vi "Check For Stop.vi"(8 "error in (no error)":errorcluster, 10 "local stop (F)":bool, 11 "User Interface in":refnum<class "User Interface.lvclass">) -> (0 "error out":errorcluster, 2 "stop?":bool, 3 "User Interface out":refnum<class "User Interface.lvclass">)   [LabVIEW 2017, in "DSF Core.lvlib" / "User Interface.lvclass"]
uses:
  User Interface.lvclass
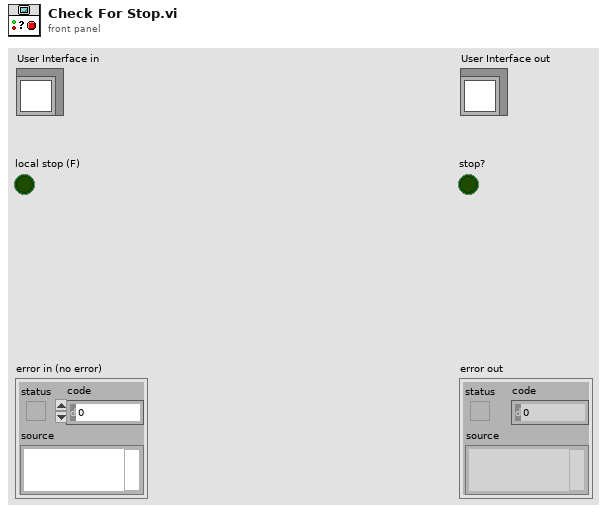
[diagram p1: front panel]
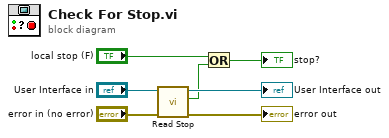
[diagram p0: block diagram]
diagram:
  n1 = call "Read Stop.vi"("error in (no error)"="error in (no error)", "User Interface in"="User Interface in") -> ("error out"=→"error out":errorcluster, "stop"=w2:bool, "User Interface out"=→"User Interface out":refnum<class "User Interface.lvclass">)  [unwired: 7 in]
  n2 = Or(x="local stop (F)", y=w2) -> (x .or. y?=→"stop?":bool)
